vi "Save_scan_as_BMP_sub_vi.vi"(8 "error in (no error)":errorcluster, 10 "Application":refnum<k7>, 11 "BMP Path In":path) -> (0 "Error Out":errorcluster, 2 "BMP":picture, 3 "BMP Path Out":path)   [LabVIEW 2016]
uses:
  <vilib>/picture/picture.llb/imagedata.ctl
panel:
  out "IsObj":bool
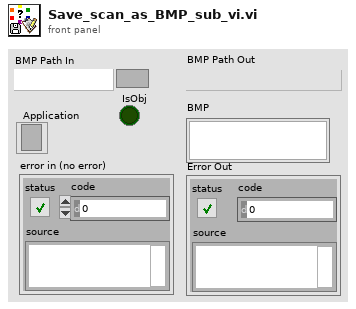
[diagram p1: front panel]
types:
  T1 = cluster{"left":i16, "top":i16, "right":i16, "bottom":i16}
  T2 = typedef "imagedata.ctl" = cluster{"image type":i32, "image depth":i32, "image":u8[], "mask":u8[], "colors":u32[], "Rectangle":cluster{"left":i16, "top":i16, "right":i16, "bottom":i16}}
  T3 = typedef "LVRectTypeDef.ctl" = cluster{"Left":i16, "Top":i16, "Right":i16, "Bottom":i16}
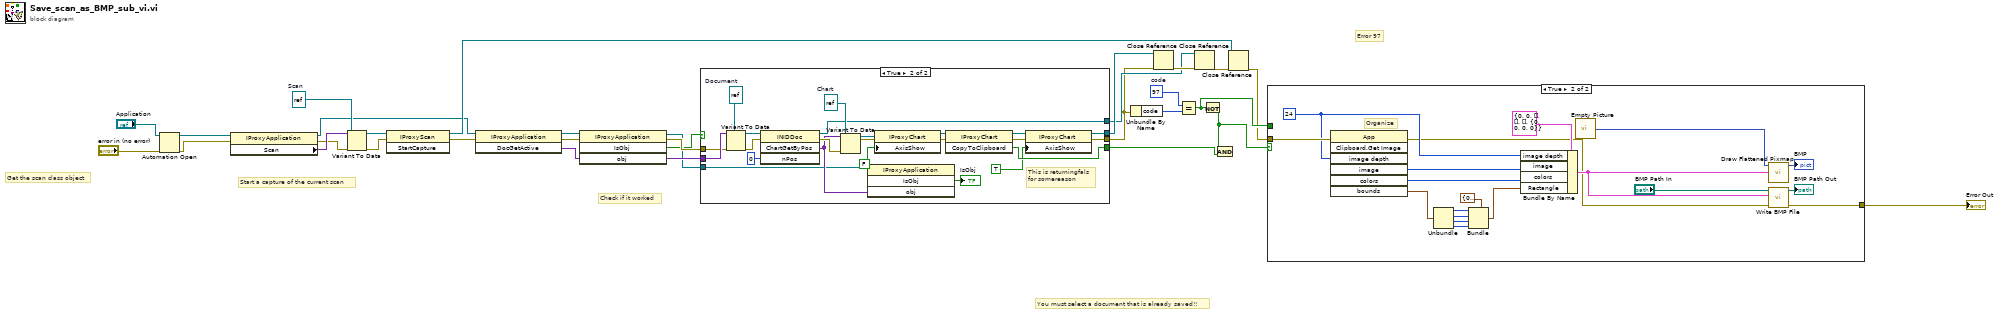
[diagram p0: block diagram]
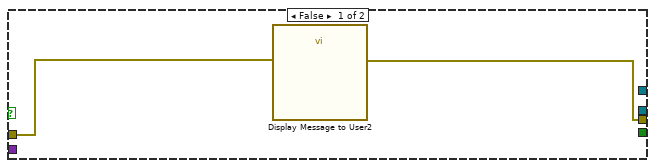
[diagram p2: hidden frame]
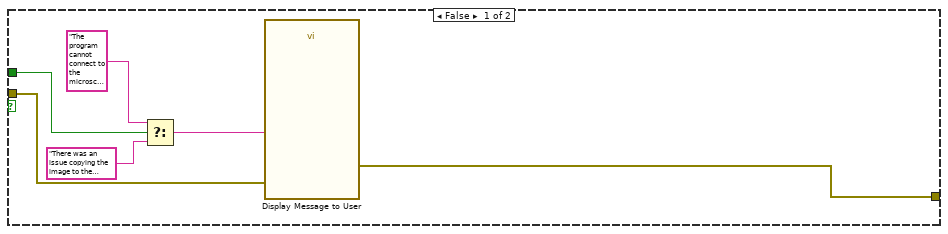
[diagram p3: hidden frame]
diagram:
  w11 = refnum<k7> refnum  # Scan
  w27 = 97  # code
  # "Check if it worked"
  # "Start a capture of the current scan"
  # "Get the scan class object"
  # "You must select a document that is already saved!!"
  # "Error 97"
  n1 = Automation Open(error in (no error)="error in (no error)", Automation Refnum="Application") -> (Automation Refnum=w14:refnum<k7>, error out=w13:errorcluster)  [unwired: 2 in]
  n2 = property class="IProxyApplication"(reference=w14, error in=w13) -> (reference out=w7:refnum<k7>, error out=w6:errorcluster, "Scan"=w17:variant)
  n3 = Variant To Data(error in=w6, type=w11, Variant=w17) -> (data=w16:refnum<k7>, error out=w15:errorcluster)
  n4 = invoke class="IProxyScan" method="StartCapture"(reference=w16, error in=w15) -> (reference out=w9:refnum<k7>, error out=w12:errorcluster)  [unwired: 1 in, 1 out]
  n5 = invoke class="IProxyApplication" method="DocGetActive"(reference=w7, error in=w12) -> (reference out=w31:refnum<k7>, error out=w28:errorcluster, "DocGetActive"=w21:variant)  [unwired: 1 in]
  n6 = invoke class="IProxyApplication" method="IsObj"(reference=w31, error in=w28, "obj"=w21) -> (reference out=w5:refnum<k7>, error out=w29:errorcluster, "IsObj"=w4:bool, "obj"=w30:variant)  [unwired: 1 in]
  n7 = case shown="True" w4 {
    tunnel: [_ w41] -> w25
    tunnel: w30 -> [_ w53]
    tunnel: w29 -> [w32 w52]
    tunnel: [w33 w42] -> w1
    tunnel: [_ w39] -> w20
    tunnel: [_ w38] -> w3
    tunnel: w5 -> [_ w35]
    frame False {
      n8 = call "Display Message to User2"("error in (no error)"=w32) -> ("error out"=w33:errorcluster)  [unwired: 9 in, 1 out]
    }
    frame True {
      w56 = refnum<k7> refnum  # Document
      w45 = refnum<k7> refnum  # Chart
      # "This is returningfals\nfor somereason"
      n9 = Variant To Data(error in=w52, type=w56, Variant=w53) -> (data=w55:refnum<k7>, error out=w54:errorcluster)
      n10 = invoke class="INIDDoc" method="ChartGetByPos"(reference=w55, error in=w54, "nPos"=0) -> (reference out=w38:refnum<k7>, error out=w51:errorcluster, "ChartGetByPos"=w37:variant)  [unwired: 1 in, 1 out]
      n11 = Variant To Data(error in=w51, type=w45, Variant=w37) -> (data=w50:refnum<k7>, error out=w47:errorcluster)
      n12 = invoke class="IProxyApplication" method="IsObj"(reference=w35, "obj"=w37) -> ("IsObj"=→"IsObj":bool)  [unwired: 2 in, 3 out]
      n13 = property class="IProxyChart"(reference=w50, error in=w47, "AxisShow"=FALSE) -> (reference out=w48:refnum<k7>, error out=w46:errorcluster)
      n14 = invoke class="IProxyChart" method="CopyToClipboard"(reference=w48, error in=w46) -> (reference out=w44:refnum<k7>, error out=w43:errorcluster, "CopyToClipboard"=w41:bool)  [unwired: 1 in]
      n15 = property class="IProxyChart"(reference=w44, error in=w43, "AxisShow"=TRUE) -> (reference out=w39:refnum<k7>, error out=w42:errorcluster)
    }
  }
  n16 = Unbundle By Name(w1) -> ("code"=w26:i32)
  n17 = Close Reference(reference=w20, error in (no error)=w1) -> (error out=w19:errorcluster)
  n18 = Equal?(x=w27, y=w26) -> (x = y?=w24:bool)
  n19 = Close Reference(reference=w3, error in (no error)=w19) -> (error out=w8:errorcluster)
  n20 = Not(x=w24) -> (.not. x?=w18:bool)
  n21 = And(x=w18, y=w25) -> ()  [unwired: 1 out]
  n22 = Close Reference(reference=w9, error in (no error)=w8) -> (error out=w2:errorcluster)
  n23 = case shown="True" w18 {
    tunnel: w2 -> [w62 w81]
    tunnel: w24 -> [w61 _]
    tunnel: [w57 w66] -> w23
    frame False {
      n24 = Select(t="The program cannot connect to the microscope API, please make sure to view the Access Codes before using the program.  If the program still does not work, then try exiting the control software, and then using  task manager to close out of the program fully.", s=w61, f="There was an issue copying the image to the clipboard, please export image manually. ") -> (s? t:f=w58:string)
      n25 = call "Display Message to User"("error in (no error)"=w62, "Message"=w58) -> ("error out"=w57:errorcluster)  [unwired: 8 in, 1 out]
    }
    frame True {
      w68 = 24 ("Image Depth")
      # "Organize"
      n26 = invoke class="App" method="Clipboard.Get Image"(error in=w81, "image depth"=w68) -> (error out=w63:errorcluster, "image"=w80:u8[], "colors"=w79:u32[], "bounds"=w71:T3)  [unwired: 5 in, 3 out]
      n27 = Unbundle(w71) -> ("Left"=w75:i16, "Top"=w74:i16, "Right"=w73:i16, "Bottom"=w72:i16)
      n28 = Bundle(cluster=T1 {"left"=0, "top"=0, "right"=0, "bottom"=0} ("Rectangle"), "left"=w75, "top"=w74, "right"=w73, "bottom"=w72) -> (w70:T1)
      n29 = Bundle By Name(cluster=T2 {"image type"=0, "image depth"=0, "image"=[], "mask"=[], "colors"=[], "Rectangle"={"left"=0, "top"=0, "right"=0, "bottom"=0}} ("image data"), "image depth"=w68, "image"=w80, "colors"=w79, "Rectangle"=w70) -> (w69:T2)
      n30 = call "Empty Picture"() -> ("empty picture"=w78:picture)
      n31 = call <vilib>:"Draw Flattened Pixmap.vi"("image data"=w69, "picture"=w78) -> ("new picture"=→"BMP":picture)  [unwired: 7 in]
      n32 = call <vilib>:"Write BMP File.vi"("error in (no error)"=w63, "image data"=w69, "path to BMP file"="BMP Path In") -> ("error out"=w66:errorcluster, "path"=→"BMP Path Out":path)  [unwired: 7 in]
    }
  }
  "Error Out" <- w23
